vi "peak comb -- interpolate -- view.vi"() -> ()   [LabVIEW 2010]
panel:
  in  "all peaks exp":i32[](array[numeric])=[564, 649, 987, 1133, 1214, 1585, 1763, 1823, 1880, 1899, 2032, 2138, 2221, 2270, 2350, 2456, 2580, 2634, 2831, 2960, 2965, 3131, 3328, 3469, 3553, 0, 3615, 3734, 0, 0, 0, 4236, 4300, 4331]
  in  "Gamma":dbl
  out "Array":dbl[](array[numeric])
  in  "freq max":dbl
  in  "freq min":dbl
  in  "df":dbl
  out "Plot: fragment":cluster{"Array":dbl[], dbl[]}(graph)
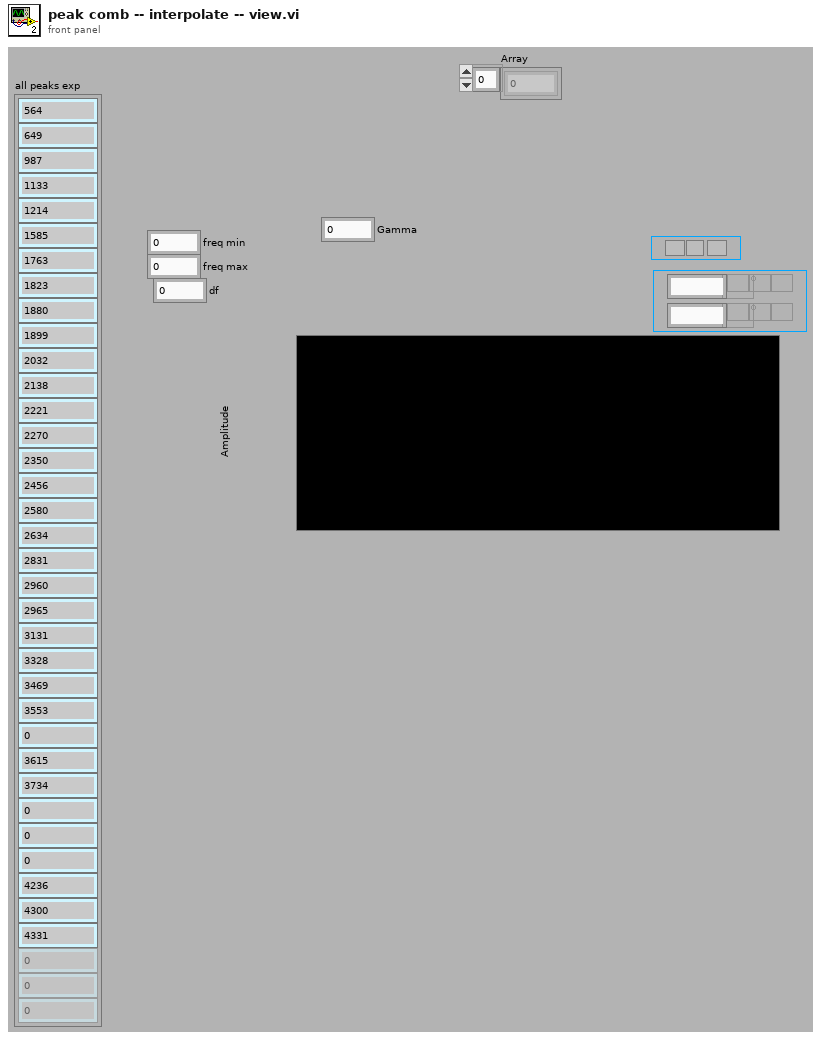
[diagram p1: front panel]
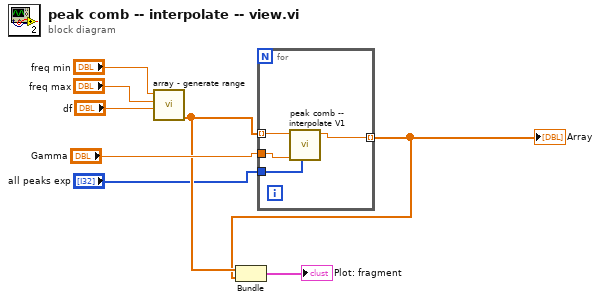
[diagram p0: block diagram]
diagram:
  n1 = call "array - generate range.vi"("df"="df", "freq max"="freq max", "freq min"="freq min") -> ("Array"=w4:dbl[])  [unwired: 8 in]
  n2 = for {
    tunnel: w4 -> [w12] mode=indexing
    tunnel: "Gamma" -> [w11]
    tunnel: [w10] -> w3 mode=indexing
    tunnel: "all peaks exp" -> [w9]
    n3 = call "peak comb -- interpolate V1.vi"("all peaks exp"=w9, "Gamma"=w11, "freq"=w12) -> ("Numeric"=w10:dbl)  [unwired: 8 in]
  }
  "Array" <- w3
  n4 = Bundle("Array"=w4, w3) -> (→"Plot: fragment":cluster{"Array":dbl[], dbl[]})  [unwired: 1 in]
